vi "DHE_DRV_add_table_entry.vi"(0 "cmd":string, 5 "type":string, 7 "dsp":string, 9 "memtype":string, 11 "error in (no error)":errorcluster, 12 "address":i32, 13 "bit":i32) -> (8 "return":i32, 15 "error out":errorcluster)   [LabVIEW 2016]
doc: "This VI turns instrument power on (Flag=1) or off (Flag=0)."
uses:
  c/lib/libarcDHE.so
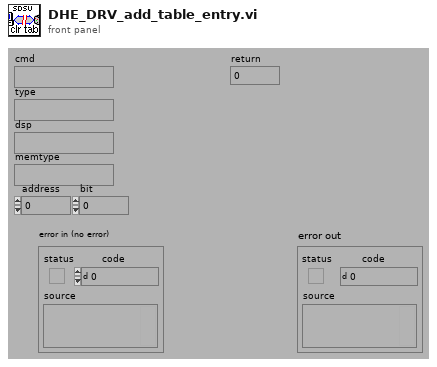
[diagram p1: front panel]
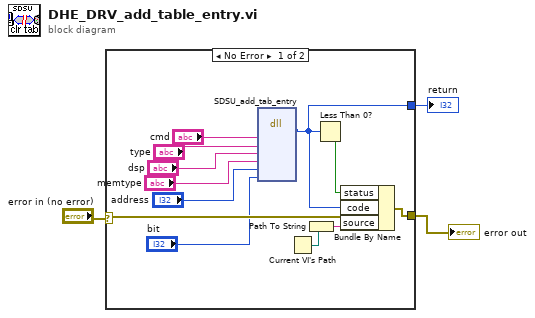
[diagram p0: block diagram]
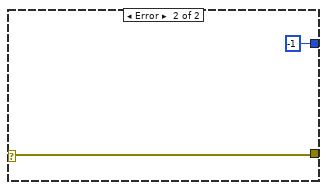
[diagram p2: hidden frame]
diagram:
  n1 = case shown="No Error" "error in (no error)" {
    selector: "error in (no error)" -> [w10 w17]
    tunnel: [w11 w17] -> w3
    tunnel: [w6 -1 ("return type")] -> w1
    frame No Error {
      n2 = dll-call lib="home/simager/panview/PAN/Modules/SDSU/private/c/lib/libarcDHE.so" fn="SDSU_add_tab_entry" label="add_table_entry"("cmd"="cmd", "type"="type", "dsp"="dsp", "memtype"="memtype", "address"="address", "bit"="bit") -> ("return type"=w6:i32)  [unwired: 9 in, 2 out]
      n3 = Current VI's Path() -> (path=w8:path)
      n4 = Path To String(path=w8) -> (string=w7:string)
      n5 = Less Than 0?(x=w6) -> (x < 0?=w9:bool)
      n6 = Bundle By Name(cluster=w10, "status"=w9, "code"=w6, "source"=w7) -> (w11:errorcluster)
    }
    frame Error {
    }
  }
  "error out" <- w3
  "return" <- w1
